vi "getPID.vi"(8 "error in (no error)":errorcluster) -> (0 "error out":errorcluster, 3 "Current PID":i64)   [LabVIEW 2013, in "ProcessInfo.lvlib"]
uses:
  ProcessInfo.lvlib
  kernel32.dll
  libc.so
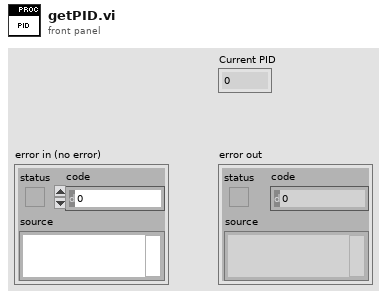
[diagram p1: front panel]
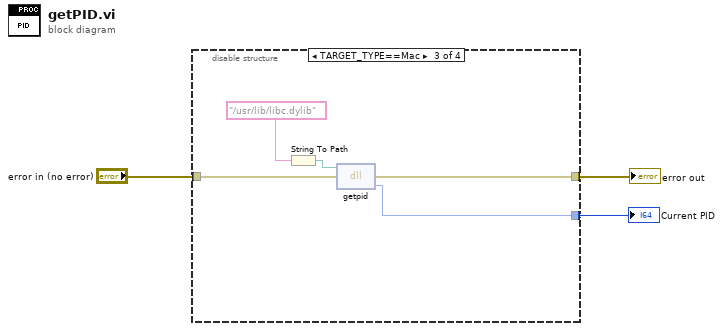
[diagram p0: block diagram]
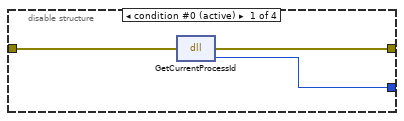
[diagram p2: hidden frame]
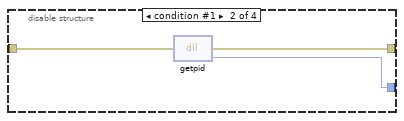
[diagram p3: hidden frame]
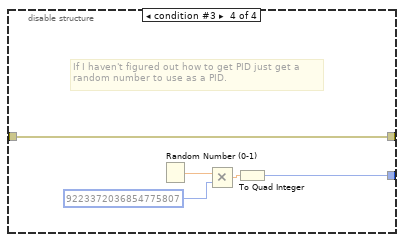
[diagram p4: hidden frame]
diagram:
  n1 = disable-structure shown="TARGET_TYPE==Mac" {
    disable-tunnel: [w6 w7 w12 w15] -> w3
    disable-tunnel: [w5 w8 w13 w19] -> w2
    disable-tunnel: "error in (no error)" -> [w4 w9 w14 w19]
    frame condition #0 (active) {
      n2 = dll-call lib="kernel32.dll" fn="GetCurrentProcessId"(error in=w4) -> (error out=w5:errorcluster, "return type"=w6:i64)  [unwired: 2 in, 1 out]
    }
    frame condition #1 {
      n3 = dll-call lib="libc.so" fn="getpid"(error in=w9) -> (error out=w8:errorcluster, "return type"=w7:i32)  [unwired: 2 in, 1 out]
    }
    frame condition #2 {
      n4 = String To Path(string="/usr/lib/libc.dylib") -> (path=w10:path)
      n5 = dll-call lib="libc.dylib" fn="getpid"(path in=w10, error in=w14) -> (error out=w13:errorcluster, "return type"=w12:u64)  [unwired: 1 in, 1 out]
    }
    frame condition #3 {
      # "If I haven't figured out how to get PID just get a\nrandom number to use as a PID."
      n6 = Random Number (0-1)() -> (number: 0 to 1=w18:dbl)
      n7 = Multiply(x=w18, y=i64 9223372036854775807 ("return type")) -> (x*y=w16:dbl)
      n8 = To Quad Integer(1:w16) -> (0:w15:i64)
    }
  }
  "Current PID" <- w3
  "error out" <- w2
